vi "Attack.vi"(8 "error in (no error)":errorcluster, 9 "Attack?":T1, 11 "Maze (0: Empty, -1: Enemy. >0: Teammate":i32[](array[numeric])) -> (0 "error out":errorcluster, 1 "Direction":i32, 2 "Action":T2, 3 "Maze (0: Empty, -1: Enemy. >0: Teammate 2":i32[](array[numeric]), 4 "Enemy Found?":bool, 6 "Enemy Direction":i32)   [LabVIEW 2014, in "Formics.lvclass"]
uses:
  Formics.lvclass
  Action Enum.ctl
  Attack Options.ctl
  SquareBattle.lvclass
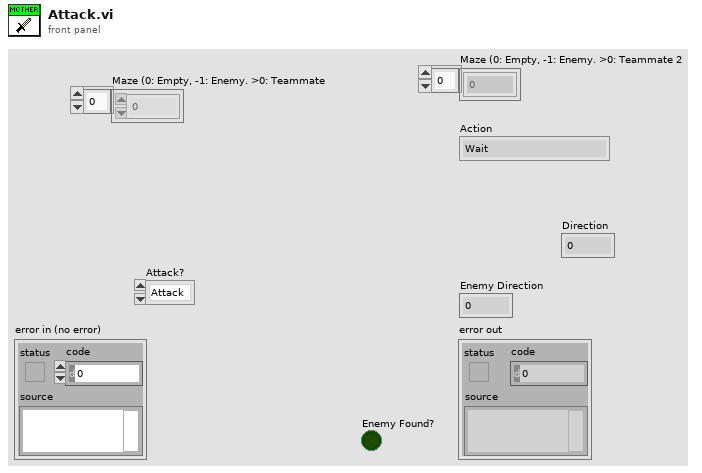
[diagram p1: front panel]
types:
  T1 = typedef "Formics.lvclass/Attack Options.ctl" = enum16{"Attack", "Run", "Distract"}
  T2 = typedef "SquareBattle.lvclass/Action Enum.ctl" = enum16{"Wait", "Move", "Attack", "Replicate"}
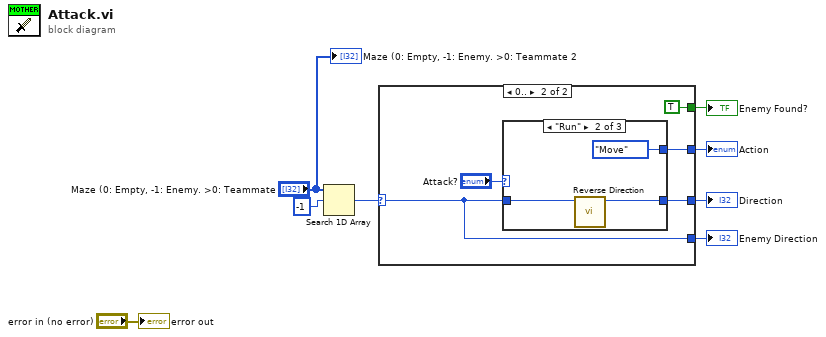
[diagram p0: block diagram]
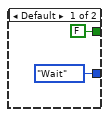
[diagram p2: hidden frame]
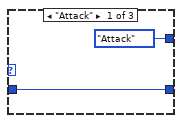
[diagram p3: hidden frame]
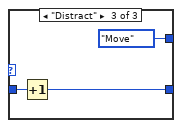
[diagram p4: hidden frame]
diagram:
  n1 = Search 1D Array(1D array="Maze (0: Empty, -1: Enemy. >0: Teammate", element=-1) -> (index of element=w2:i32)  [unwired: 1 in]
  n2 = case shown="0.." w2 {
    selector: w2 -> [_ w11]
    tunnel: [Action_Enum."Wait" ("Action") w15] -> w6
    tunnel: [_ w13] -> w7
    tunnel: [FALSE ("Enemy Found?") TRUE ("Enemy Found?")] -> w3
    tunnel: [_ w11] -> w1
    frame Default {
    }
    frame 0.. {
      n3 = case shown="\"Run\"" "Attack?" {
        tunnel: [Action_Enum."Attack" ("Action") Action_Enum."Move" ("Action") Action_Enum."Move" ("Action")] -> w15
        tunnel: [w16 w18 w21] -> w13
        tunnel: w11 -> [w16 w19 w22]
        frame "Attack" {
        }
        frame "Run" {
          n4 = call "Reverse Direction.vi"("Direction"=w19) -> ("Numeric"=w18:i32)  [unwired: 10 in]
        }
        frame "Distract" {
          n5 = Increment(x=w22) -> (x+1=w21:i32)
        }
      }
    }
  }
  "Action" <- w6
  "Direction" <- w7
  "Enemy Found?" <- w3
  "Enemy Direction" <- w1
  "error out" <- "error in (no error)"
  "Maze (0: Empty, -1: Enemy. >0: Teammate 2" <- "Maze (0: Empty, -1: Enemy. >0: Teammate"
